vi "BinRemovalSelector.vi"(8 "error in (no error)":errorcluster, 10 "Lower Bounds":dbl[](array[numeric]), 11 "Upper Bounds":dbl[](array[numeric])) -> (0 "error out":errorcluster, 2 "RemoveLowestBin":bool, 3 "RemoveHighestBin":bool)   [LabVIEW 2012, in "Histogram Custom Device.lvlib"]
uses:
  Histogram Custom Device.lvlib
panel:
  out "Highest Bin":string
  out "Lowest Bin":string
  in  "Remove Highest Bin?":bool
  in  "Remove Lowest Bin?":bool
  in  "Done?":bool
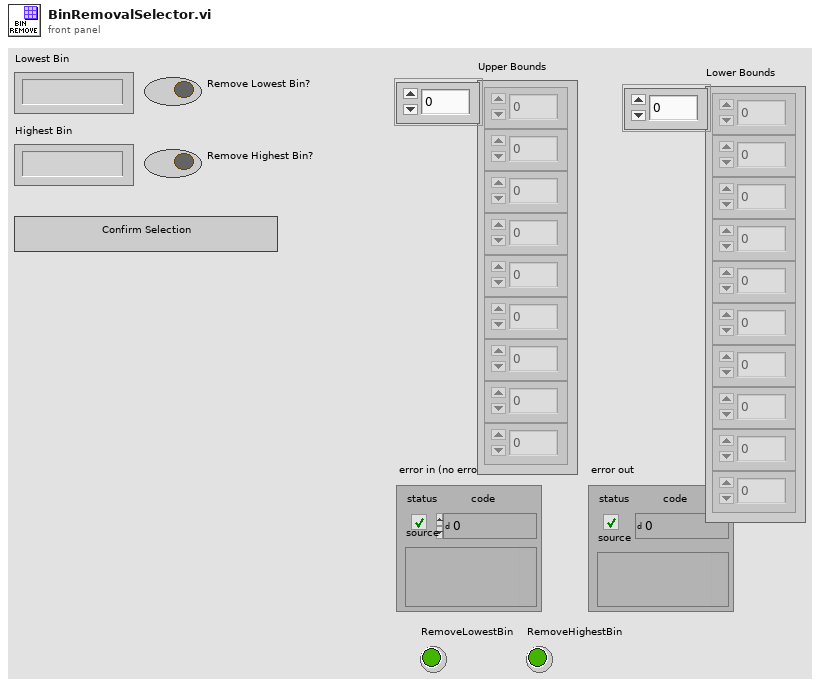
[diagram p1: front panel]
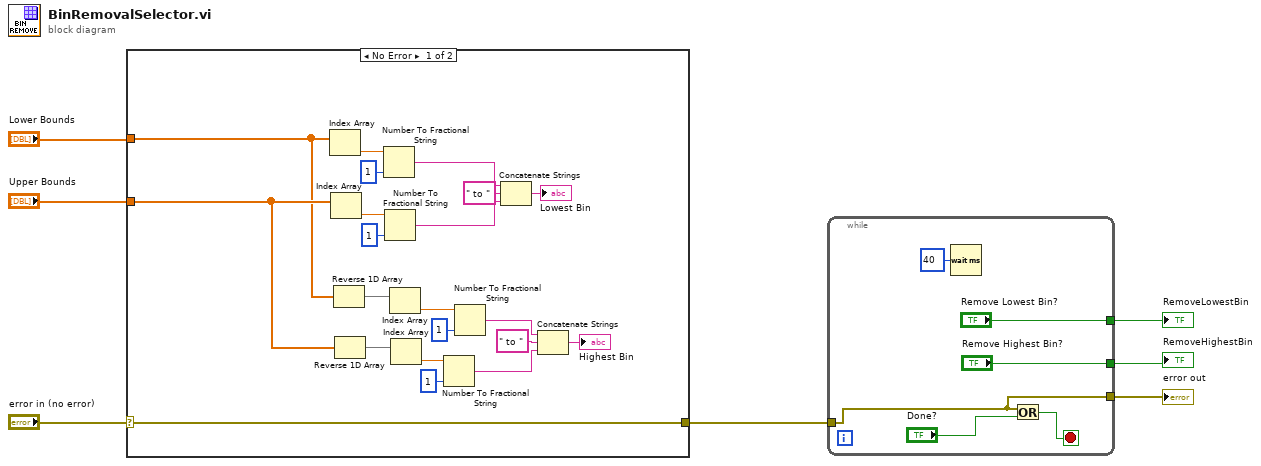
[diagram p0: block diagram]
diagram:
  n1 = case shown="No Error" "error in (no error)" {
    selector: "error in (no error)" -> [w10 w29]
    tunnel: [w10 w29] -> w6
    tunnel: "Upper Bounds" -> [w9 _]
    tunnel: "Lower Bounds" -> [w8 _]
    frame No Error {
      n2 = Index Array(array=w8) -> (element=w14:dbl)  [unwired: 1 in]
      n3 = Index Array(array=w9) -> (element=w11:dbl)  [unwired: 1 in]
      n4 = Reverse 1D Array(array=w8) -> (reversed array=w27:dbl[])
      n5 = Reverse 1D Array(array=w9) -> (reversed array=w26:dbl[])
      n6 = Number To Fractional String(number=w14, precision (6)=i16 1) -> (F-format string=w16:string)  [unwired: 2 in]
      n7 = Number To Fractional String(number=w11, precision (6)=i16 1) -> (F-format string=w17:string)  [unwired: 2 in]
      n8 = Index Array(array=w27) -> (element=w28:dbl)  [unwired: 1 in]
      n9 = Index Array(array=w26) -> (element=w25:dbl)  [unwired: 1 in]
      n10 = Number To Fractional String(number=w25, precision (6)=i16 1) -> (F-format string=w20:string)  [unwired: 2 in]
      n11 = Number To Fractional String(number=w28, precision (6)=i16 1) -> (F-format string=w21:string)  [unwired: 2 in]
      n12 = Concatenate Strings(w16, " to " ("string"), w17) -> (→"Lowest Bin":string)
      n13 = Concatenate Strings(w21, " to " ("string"), w20) -> (→"Highest Bin":string)
    }
    frame Error {
    }
  }
  n14 = while {
    tunnel: w6 -> [w32]
    tunnel: [w32] -> w3
    tunnel: ["Remove Lowest Bin?"] -> w2
    tunnel: ["Remove Highest Bin?"] -> w1
    stop <- w34 stop-if-true
    n15 = Wait (ms)(milliseconds to wait=u32 40) -> ()  [unwired: 1 out]
    n16 = Or(x=w32, y="Done?") -> (x .or. y?=w34:bool)
  }
  "error out" <- w3
  "RemoveHighestBin" <- w1
  "RemoveLowestBin" <- w2
